vi "Header Valid.vi"(8 "eof on previous":bool, 9 "input valid":bool, 11 "input data":bool[](array[boolean])) -> (0 "expected":bool, 1 "header detected":bool, 2 "timestamp":u64, 3 "chdr_header":T1)   [LabVIEW 2023, in "CHDR Support.lvlib"]
doc: "Detects and parses packet headers and optionally can determine if the header was expected."
uses:
  CHDR Support.lvlib
  CHDR Header Layout.ctl
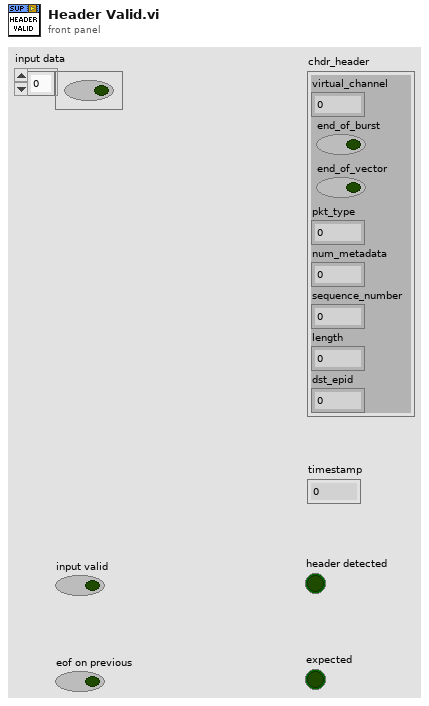
[diagram p1: front panel]
types:
  T1 = typedef "CHDR Support.lvlib/CHDR Header Layout.ctl" = cluster{"virtual_channel":fxp<+,6,6>, "end_of_burst":bool, "end_of_vector":bool, "pkt_type":fxp<+,3,3>, "num_metadata":fxp<+,5,5>, "sequence_number":u16, "length":u16, "dst_epid":u16}
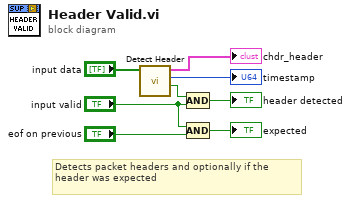
[diagram p0: block diagram]
diagram:
  # "Detects packet headers and optionally if the header was expected"
  n1 = call "Detect Header.vi"("input data"="input data") -> ("header detected"=w5:bool, "timestamp"=→"timestamp":u64, "chdr_header"=→"chdr_header":T1)  [unwired: 8 in]
  n2 = Compound Arithmetic op=AND(w5, "input valid") -> (→"header detected":bool)
  n3 = Compound Arithmetic op=AND("input valid", "eof on previous") -> (→"expected":bool)
